vi "Insert Error.Record_New.vi"(7 "Code":string, 8 "error in (no error)":errorcluster, 9 "Source":string, 10 "Case":string, 11 "Model":string) -> (0 "error out":errorcluster)   [LabVIEW 2017, in "SQLite.lvclass"]
doc: "更新Limitation表格里面的Min和Max，根据输入的不同而更新不同的内容。\nValue 的输入必须最少包含Min和Max的值。\n\n2015-11-03 10:20:20\n蒋松\njiangsong@outlook.com"
uses:
  SQLite.lvclass
  SQLiteFileName.ctl
  TabelFullName.ctl
  <vilib>/Utility/error.llb/Trim Whitespace.vi
  <userlib>/sushu/sushu.lvlib
  <userlib>/LabSQL/LabSQL.lvlib
panel:
  in  "VI Ref":refnum<vi>
  in  "Alarm?":bool=TRUE
  in  "CMD":T1(ring)=enum."Read"
  out "concatenated string":string
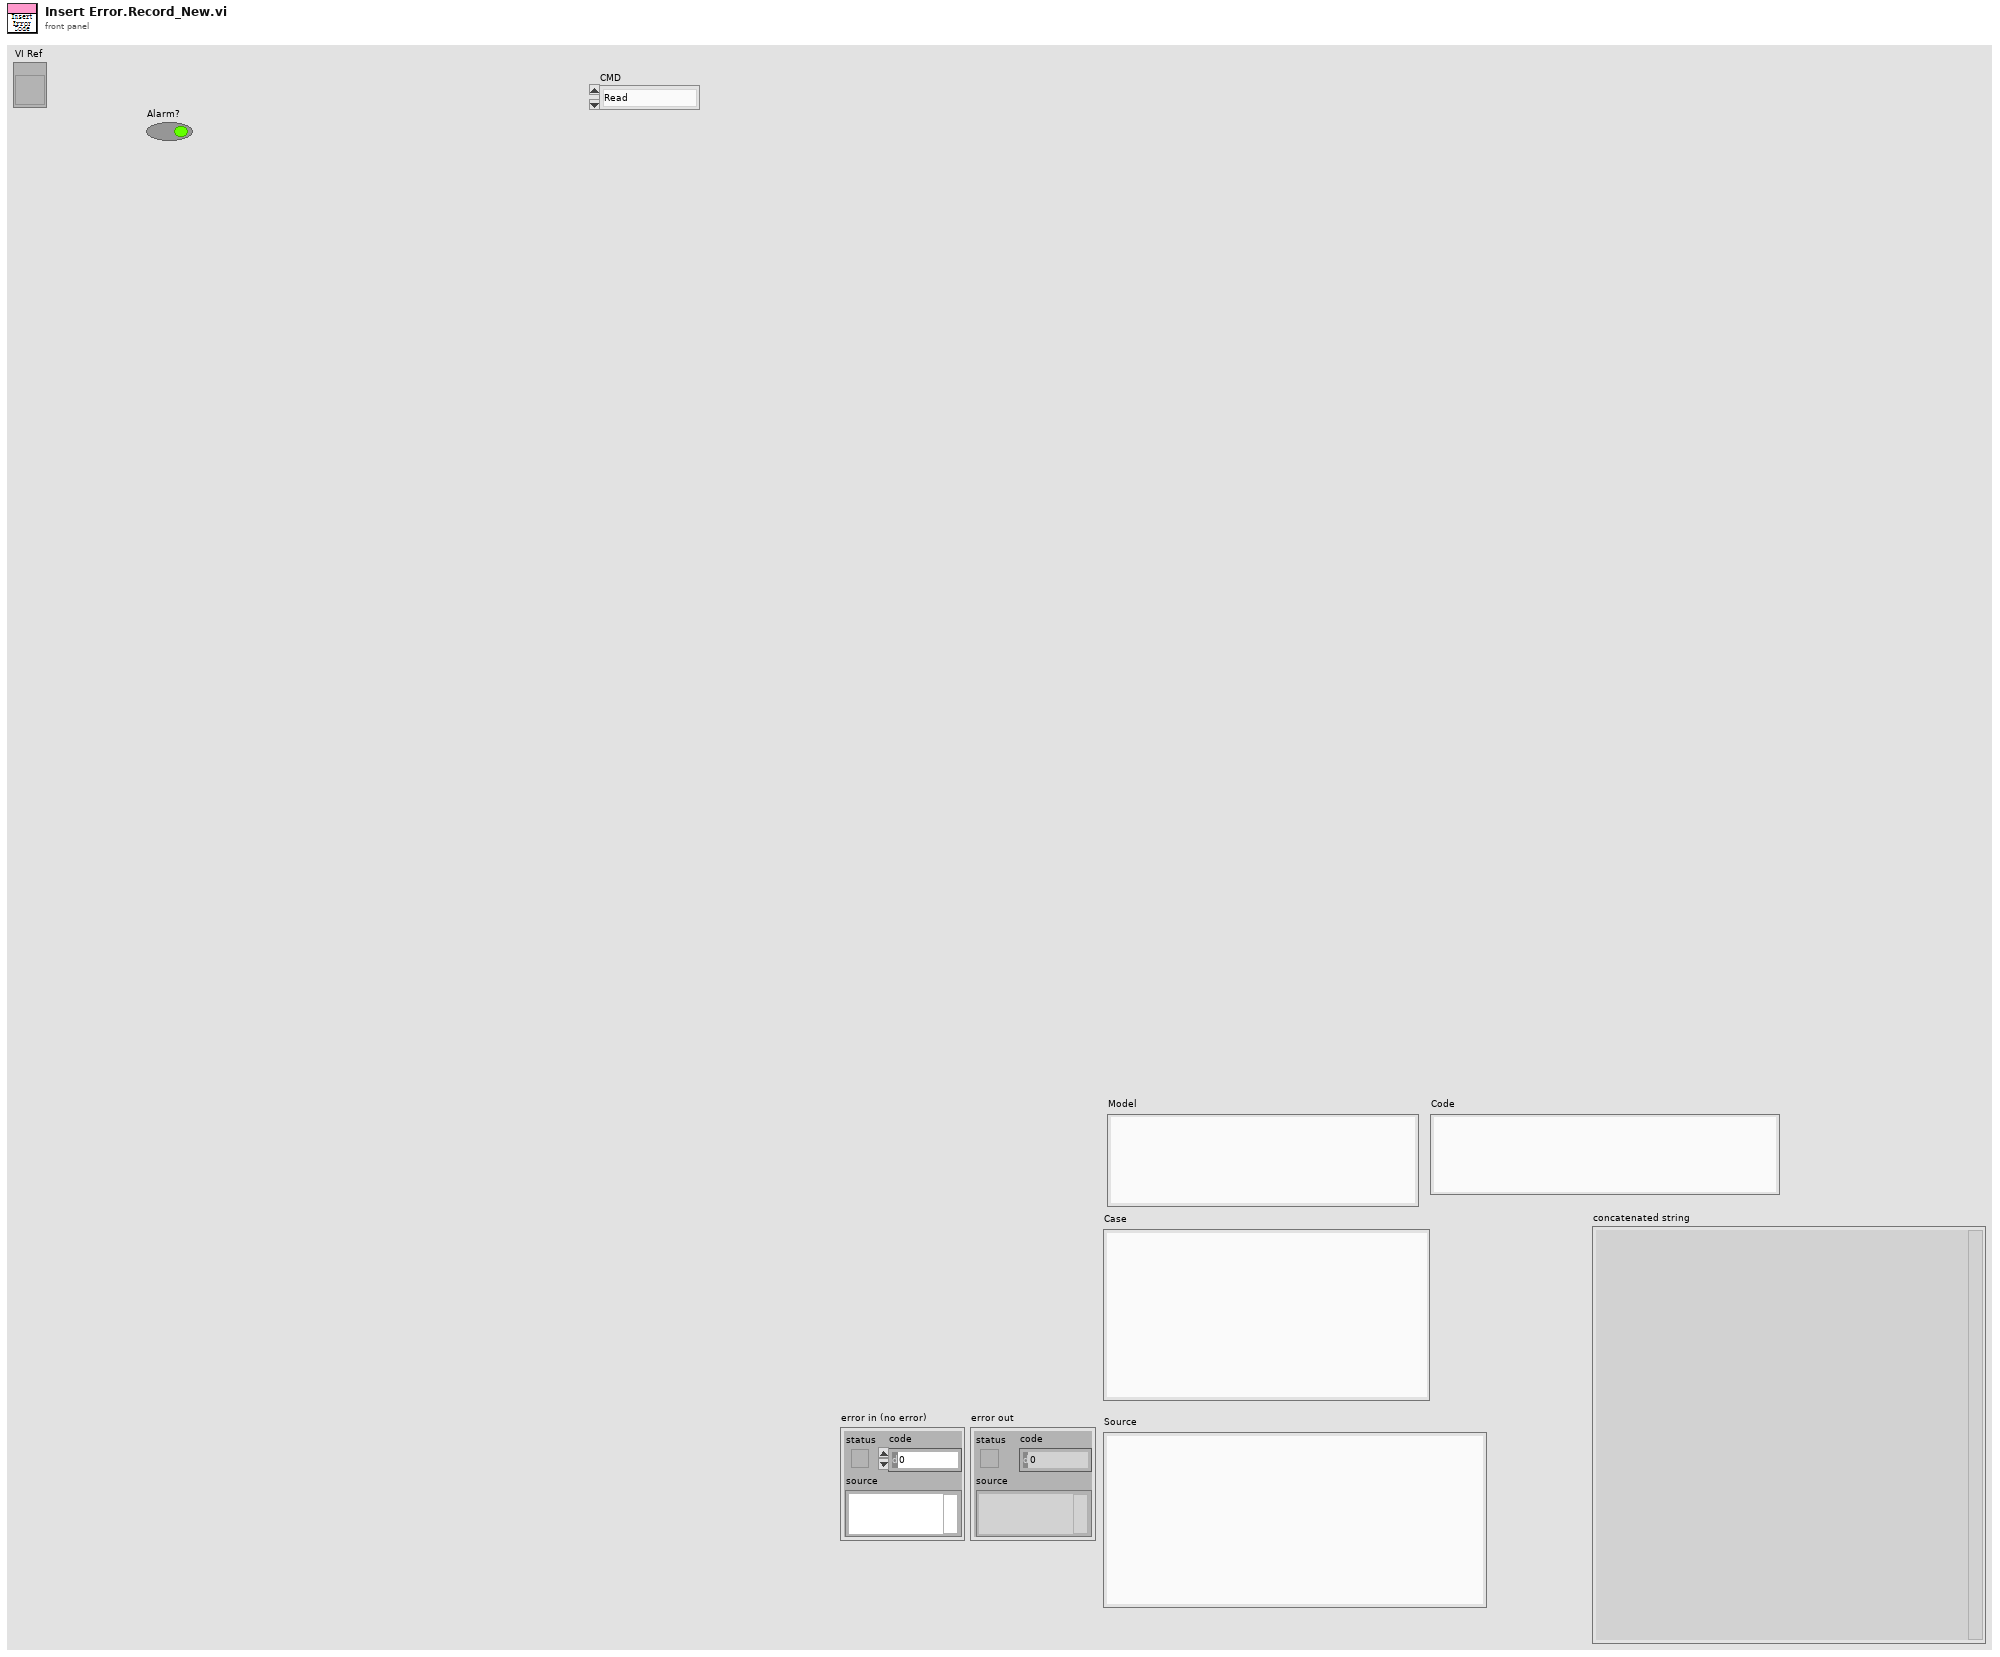
[diagram p1: front panel]
types:
  T1 = enum16{"Initialize", "Read", "Write", "UnInitialize"}
  T2 = typedef "SQLite.lvclass/TabelFullName.ctl" = string
  T3 = typedef "SQLite.lvclass/SQLiteFileName.ctl" = string
  T4 = cluster{"Current VI Reference":refnum<vi>, "Close Panel on Exit?":bool}
  T5 = cluster{"Core":cluster{"Current VI Reference":refnum<vi>, "Close Panel on Exit?":bool}, "VI Name":string}
  T6 = enum32{"invalid app kind", "Development System", "Run Time System", "Student Edition", "Embedded LabVIEW", "Evaluation", "Custom"}
  T7 = enum32{"Invalid", "Standard", "Closed", "Hidden", "Minimized", "Maximized"}
  T8 = enum16{"Other", "SQL2008", "SQLite", "Access", "MySQL"}
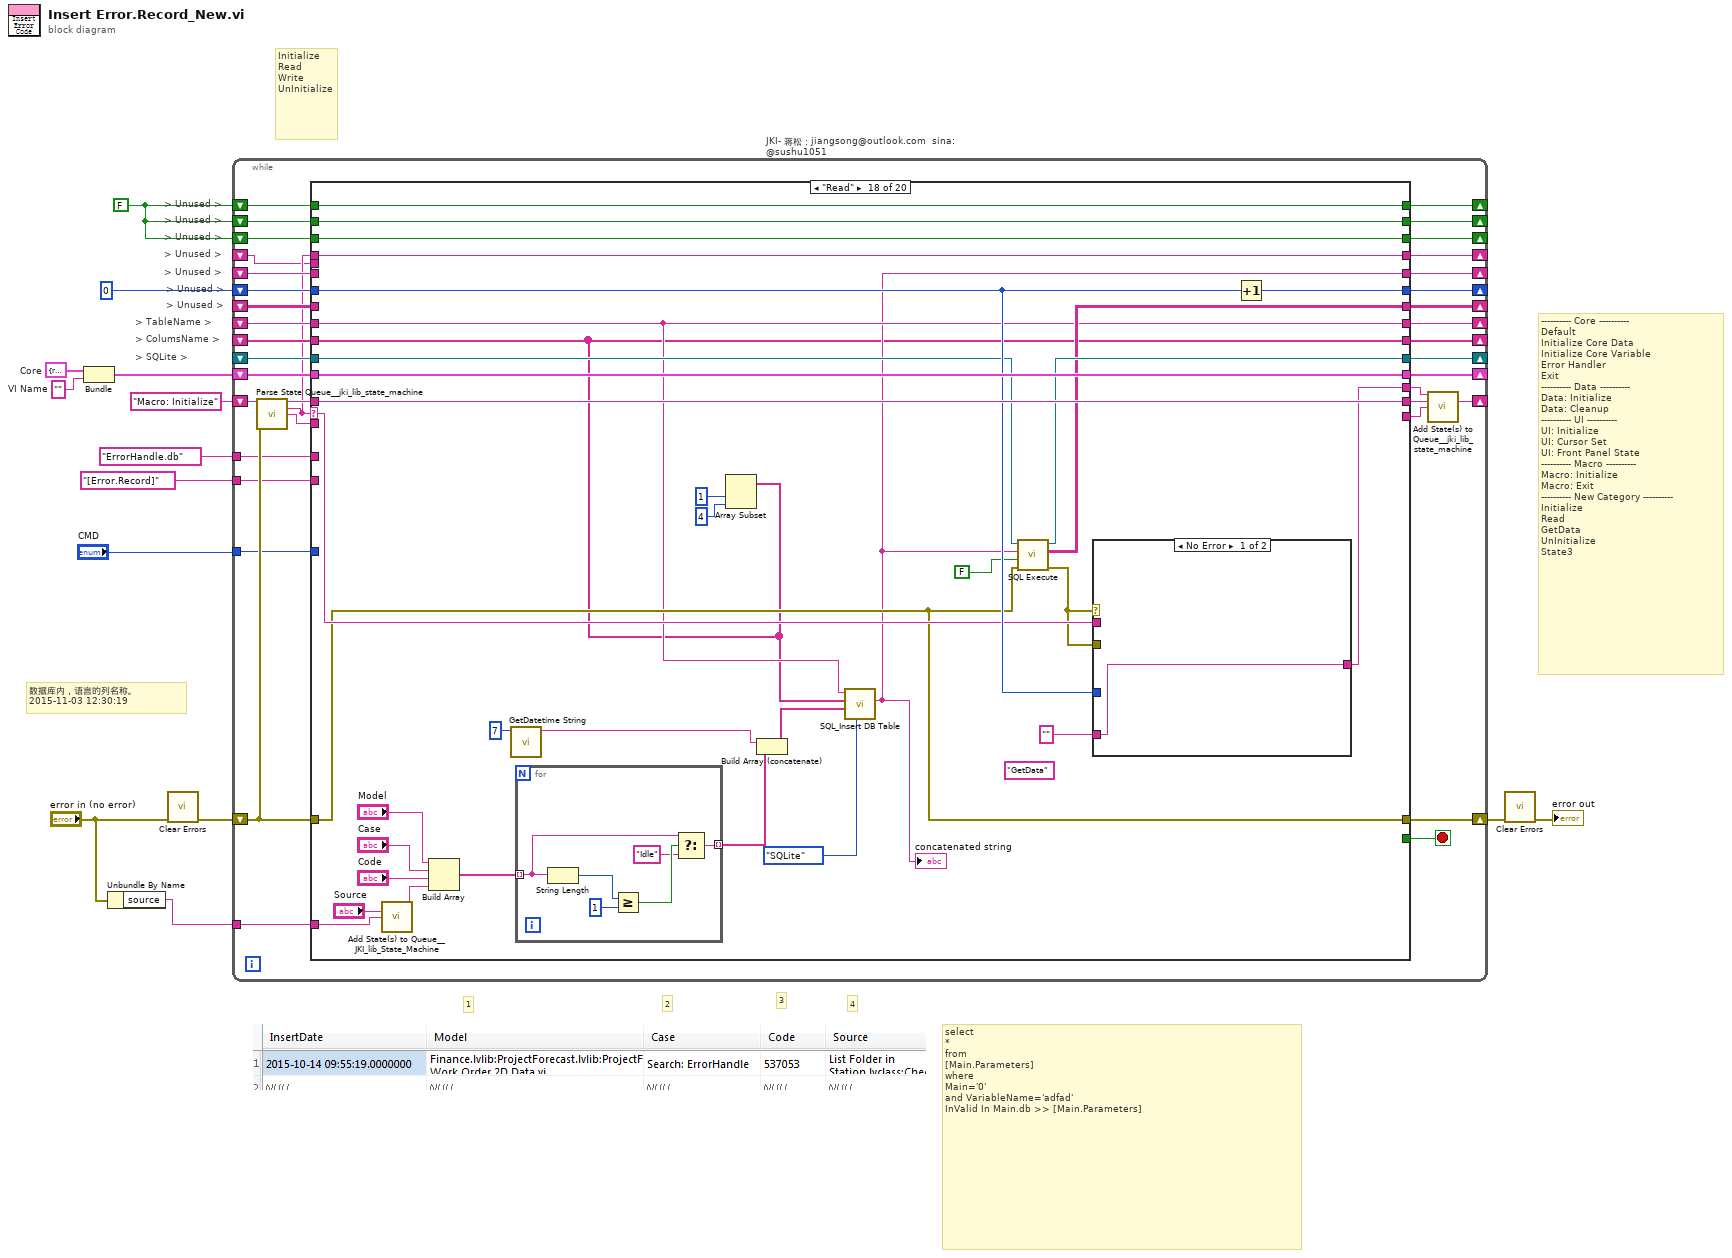
[diagram p0: block diagram]
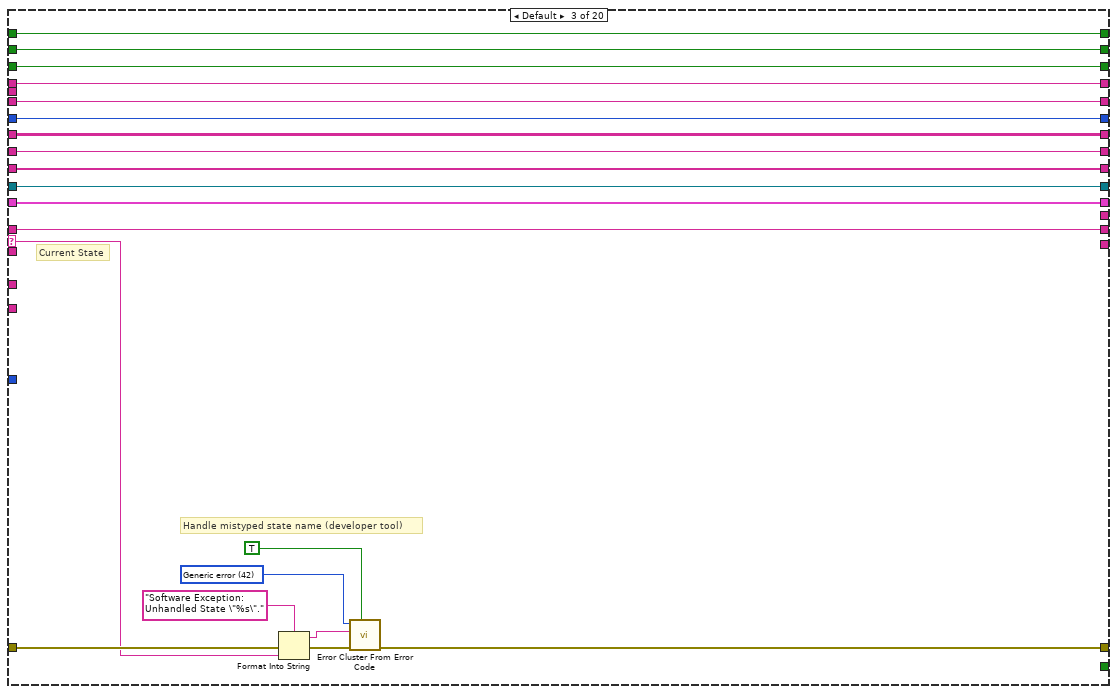
[diagram p4: hidden frame]
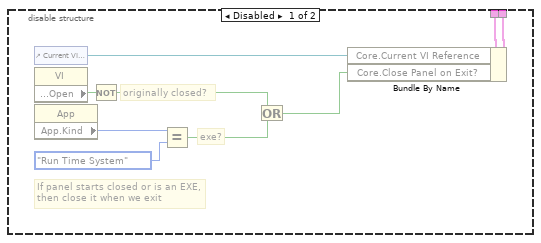
[diagram p6: hidden frame]
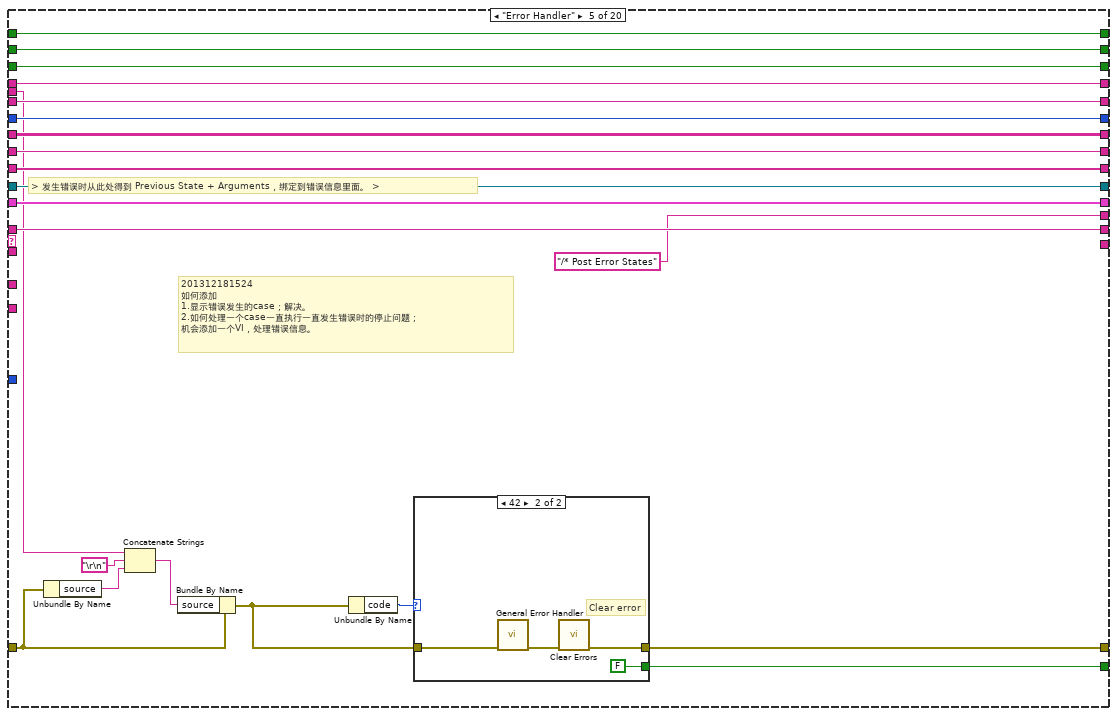
[diagram p7: hidden frame]
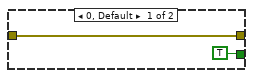
[diagram p8: hidden frame]
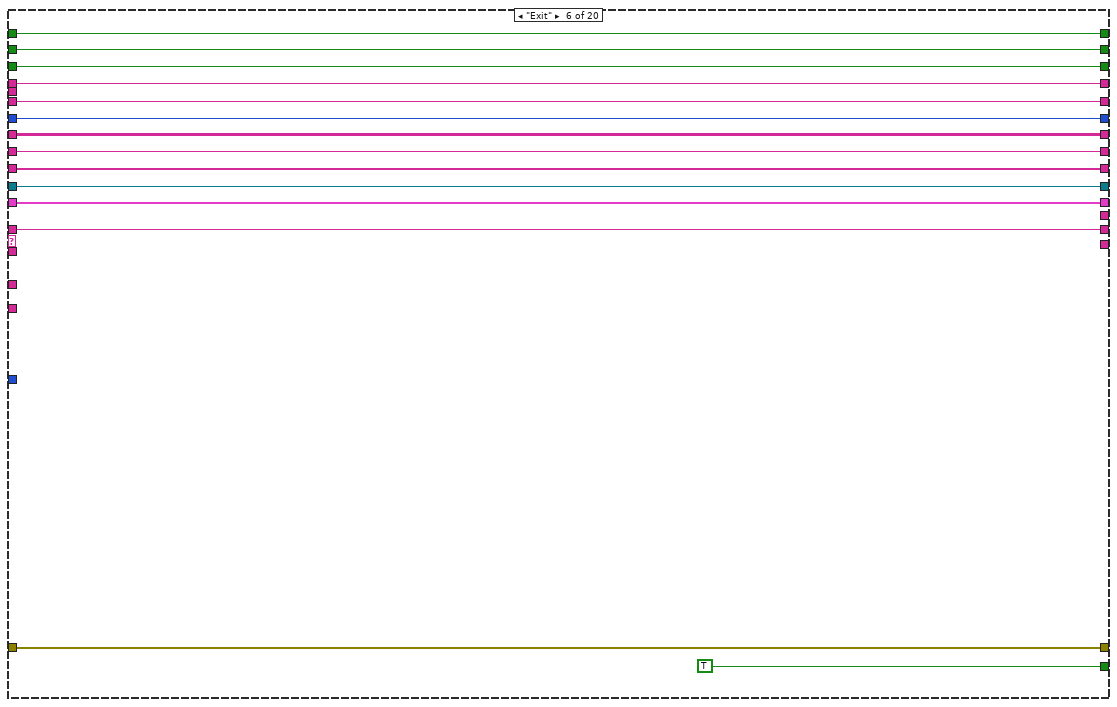
[diagram p9: hidden frame]
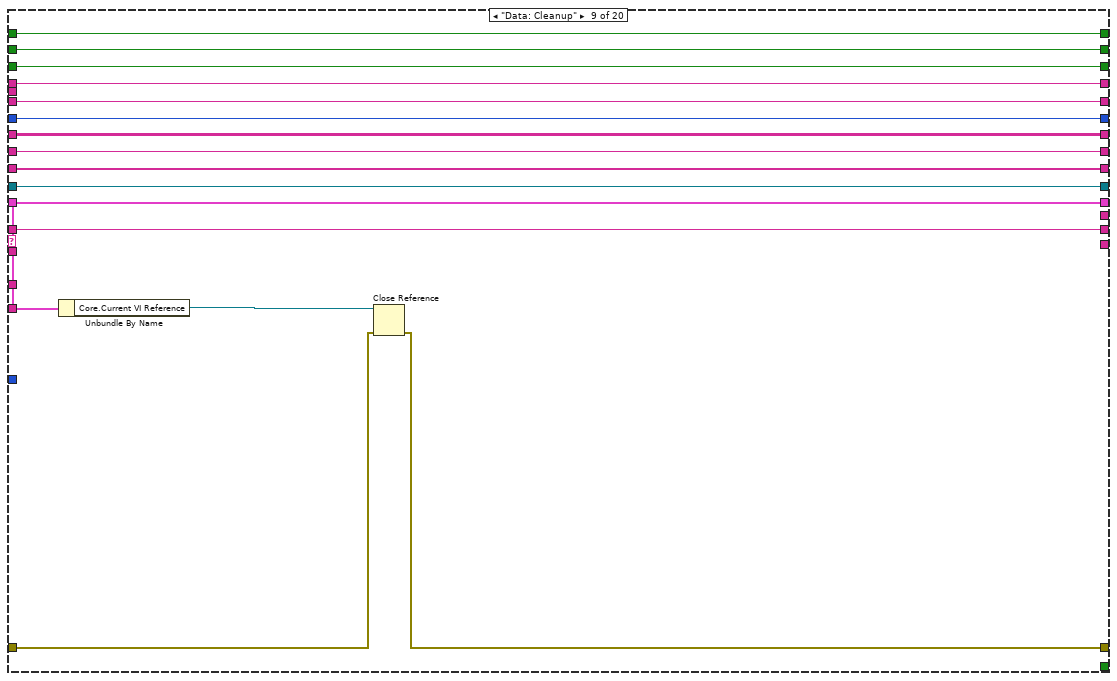
[diagram p12: hidden frame]
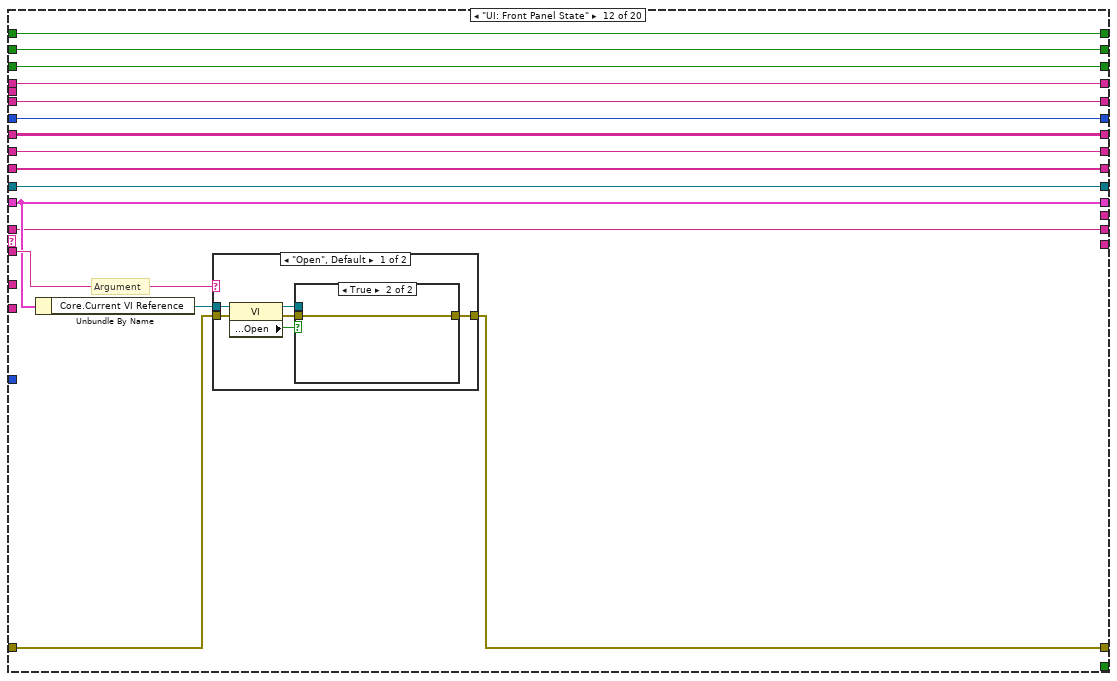
[diagram p15: hidden frame]
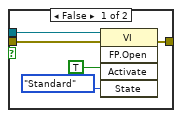
[diagram p16: hidden frame]
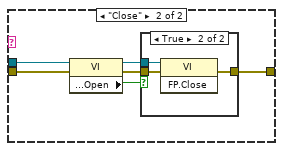
[diagram p17: hidden frame]
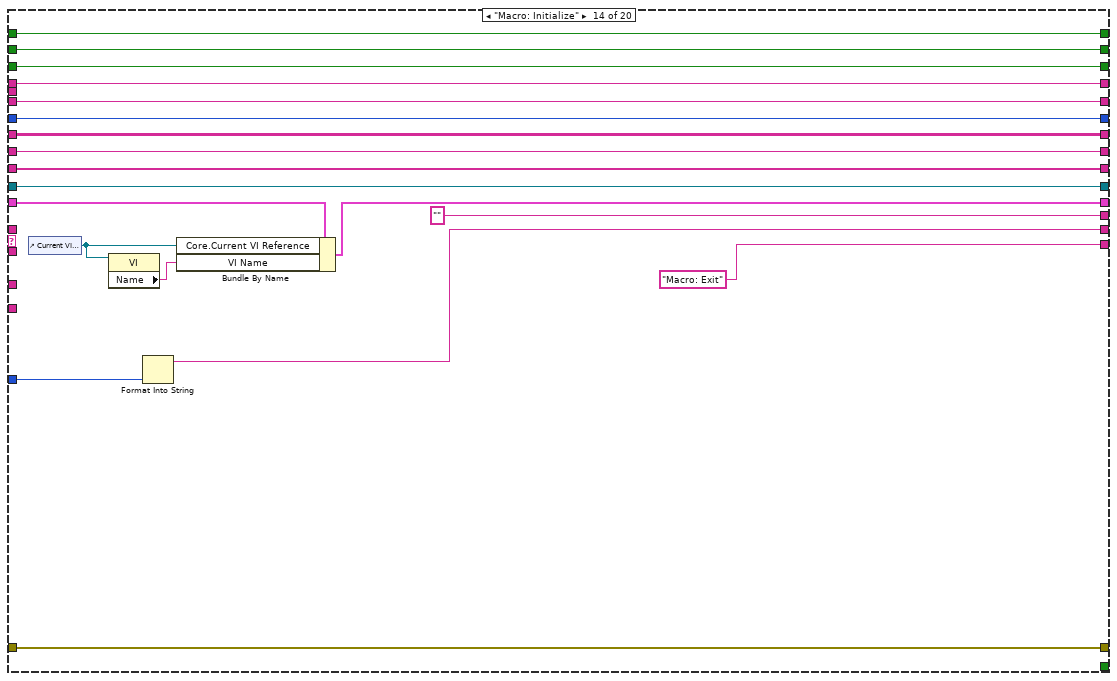
[diagram p20: hidden frame]
diagram:
  w14 = ""  # VI Name
  w13 = T4 {"Current VI Reference"=refnum, "Close Panel on Exit?"=FALSE}  # Core
  w8 = FALSE
  # "Initialize\nRead\nWrite\nUnInitialize"
  # "> Unused >"
  # "> Unused >"
  # "> Unused >"
  # "> Unused >"
  # "> Unused >"
  # "> Unused >"
  # "> SQLite >"
  # "> ColumsName >"
  # "> TableName >"
  # "> Unused >"
  # "---------- Core ----------\nDefault\nInitialize Core Data\nInitialize Core Variable\nError Handler\nExit\n---------- Data ----------\nData: Initialize\nData: Cleanup\n---------- UI ----------\nUI: Initialize\nUI: Cursor Set\nUI: Front Panel State\n---------- Macro ----------\nMacro: Initialize\nMacro: Exit\n---------- New Category ----------\nInitialize\nRead\nGetData\nUnInitialize\nState3"
  # "数据库内，语言的列名称。\n2015-11-03 12:30:19"
  # "4"
  # "3"
  # "2"
  # "1"
  # "select\n*\nfrom\n[Main.Parameters]\nwhere\nMain='0'\nand VariableName='adfad'\nInValid In Main.db >> [Main.Parameters]"
  n1 = Bundle("Core"=w13, "VI Name"=w14) -> (w12:T5)  [unwired: 1 in]
  n2 = Unbundle By Name("error in (no error)") -> ("source"=w2:string)
  n3 = call <vilib>:"Clear Errors.vi"("error in (no error)"="error in (no error)") -> ("error out"=w4:errorcluster)  [unwired: 5 in, 1 out]
  n4 = while "JKI- 蒋松：jiangsong@outlook.com  sina: @sushu1051" {
    shift-right: [w49] -> w5
    shift-left: w4 -> [w47]
    shift-right: [w36] -> _
    shift-left: "Macro: Initialize" -> [w37]
    shift-right: [w43] -> _
    shift-left: _ -> [w45]
    shift-right: [w44] -> _
    shift-left: _ -> [w46]
    shift-right: [w38] -> _
    shift-left: w12 -> [w41]
    shift-right: [w39] -> _
    shift-left: _ -> [w32]
    shift-right: [w40] -> _
    shift-left: _ -> [w42]
    shift-right: [w31] -> _
    shift-left: 0 -> [w30]
    shift-right: [w24] -> _
    shift-left: w8 -> [w22]
    shift-right: [w23] -> _
    shift-left: w8 -> [w21]
    shift-right: [w26] -> _
    shift-left: _ -> [w27]
    shift-right: [w25] -> _
    shift-left: _ -> [w16]
    shift-right: [w28] -> _
    shift-left: w8 -> [w29]
    tunnel: "CMD" -> [w20]
    tunnel: T3 "ErrorHandle.db" ("SQLiteFileName") -> [w19]
    tunnel: T2 "[Error.Record]" ("TabelFullName") -> [w18]
    tunnel: w2 -> [w15]
    stop <- w48 stop-if-true
    n5 = call <vilib>:"Parse State Queue__jki_lib_state_machine.vi"("State Queue"=w37, "Error In (no error)"=w47) -> ("Remaining States"=w51:string, "Current State"=w17:string, "Arguments"=w50:string)  [unwired: 10 in, 1 out]
    n6 = case shown="\"Read\"" w17 {
      selector: w17 -> [_ _ w85 _ _ _ _ _ _ _ _ _ _ _ _ _ _ w375 _ _]
      tunnel: w51 -> [w64 w71 w84 w104 w135 w156 w170 w184 w196 w211 w224 w237 w275 _ w308 w325 w351 w385 w421 w454]
      tunnel: w50 -> [_ _ _ _ _ _ _ _ _ _ _ w240 _ _ _ _ _ _ _ _]
      tunnel: [w63 w77 w86 w108 w129 w158 w172 w186 w198 w213 w226 w241 w277 w297 w315 w328 w332 w371 w406 w440] -> w49
      tunnel: w47 -> [w63 w77 w87 w108 w139 w158 w172 w186 w199 w213 w226 w242 w277 w297 w315 w328 w332 w371 w407 w441]
      tunnel: [w64 w71 w84 w104 w135 w156 w170 w184 w196 w211 w224 w237 w275 w283 w308 w325 w351 w385 w421 w454] -> w35
      tunnel: [_ _ _ _ w128 TRUE _ _ _ _ _ _ _ _ _ _ _ _ _ _] -> w48
      tunnel: w46 -> [w62 w76 w97 w111 w143 w163 w176 w189 w204 w217 w230 w246 w281 w300 w318 w331 w350 _ w408 w453]
      tunnel: w45 -> [w61 w75 w96 w110 w142 w162 w175 w188 w203 w216 w229 w245 w280 w299 w317 w330 _ w367 w420 w452]
      tunnel: [w62 w76 w97 w111 w143 w163 w176 w189 w204 w217 w230 w246 w281 w300 w318 w331 w350 w372 w408 w453] -> w44
      tunnel: [w61 w75 w96 w110 w142 w162 w175 w188 w203 w216 w229 w245 w280 w299 w317 w330 w333 w367 w420 w452] -> w43
      tunnel: w42 -> [w60 w74 w95 w109 w141 w161 w174 w187 w202 w215 w228 w244 w279 w298 w316 w329 _ w356 w419 w451]
      tunnel: w32 -> [w58 w72 w94 w105 w133 w157 w171 w185 w197 w212 w225 w238 w276 w296 w309 w326 _ w374 w418 w443]
      tunnel: w41 -> [w59 w73 w93 w107 w140 w160 w173 w177 w200 w214 w227 w239 w278 w285 w310 w327 w349 w384 w417 w450]
      tunnel: [w60 w74 w95 w109 w141 w161 w174 w187 w202 w215 w228 w244 w279 w298 w316 w329 w335 w356 w419 w451] -> w40
      tunnel: [w58 w72 w94 w105 w133 w157 w171 w185 w197 w212 w225 w238 w276 w296 w309 w326 w337 w373 w418 w442] -> w39
      tunnel: [w59 w73 w93 w106 w140 w160 w173 w177 w200 w214 w227 w239 w278 w284 w310 w327 w349 w384 w417 w450] -> w38
      tunnel: [_ _ _ _ "/* Post Error States" _ _ _ _ _ _ _ _ "" w307 _ _ w377 _ _] -> w34
      tunnel: [_ _ _ _ _ _ _ _ _ _ _ _ _ "Macro: Exit" _ _ _ _ _ _] -> w33
      tunnel: w30 -> [w57 w70 w83 w103 w132 w155 w169 w183 w195 w210 w223 w236 w274 w295 w306 w324 w348 w378 w416 w449]
      tunnel: [w57 w70 w83 w103 w132 w155 w169 w183 w195 w210 w223 w236 w274 w295 w306 w324 w348 w379 w416 w449] -> w31
      tunnel: w21 -> [w55 w68 w81 w101 w126 w153 w167 w181 w193 w208 w221 w234 w272 w291 w304 w322 w343 w382 w415 w448]
      tunnel: w22 -> [w54 w67 w80 w100 w125 w152 w166 w180 w192 w207 w220 w233 w271 w290 w303 w321 w344 w381 w414 w447]
      tunnel: [w55 w68 w81 w101 w126 w153 w167 w181 w193 w208 w221 w234 w272 w291 w304 w322 w343 w382 w415 w448] -> w23
      tunnel: [w54 w67 w80 w100 w125 w152 w166 w180 w192 w207 w220 w233 w271 w290 w303 w321 w344 w381 w414 w447] -> w24
      tunnel: w17 -> [w53 w66 w79 w99 w124 w151 w165 w179 w191 w206 w219 w232 w270 w289 w302 w320 w345 w380 w413 w446]
      tunnel: w27 -> [w52 w65 w78 w98 w123 w150 w164 w178 w190 w205 w218 w231 w269 w288 w301 w319 w346 _ w403 w445]
      tunnel: [w53 w66 w79 w99 w124 w151 w165 w179 w191 w206 w219 w232 w270 w289 w302 w320 w345 w380 w413 w446] -> w25
      tunnel: [w52 w65 w78 w98 w123 w150 w164 w178 w190 w205 w218 w231 w269 w288 w301 w319 w346 w366 w403 w445] -> w26
      tunnel: w29 -> [w56 w69 w82 w102 w127 w154 w168 w182 w194 w209 w222 w235 w273 w292 w305 w323 w347 w383 w412 w444]
      tunnel: [w56 w69 w82 w102 w127 w154 w168 w182 w194 w209 w222 w235 w273 w292 w305 w323 w347 w383 w412 w444] -> w28
      tunnel: w20 -> [_ _ _ _ _ _ _ _ _ _ _ _ _ w282 _ _ _ _ _ _]
      tunnel: w19 -> [_ _ _ _ _ _ _ _ _ _ _ _ _ _ _ _ w336 _ w405 _]
      tunnel: w18 -> [_ _ _ _ _ _ _ _ _ _ _ _ _ _ _ _ w334 _ w404 _]
      tunnel: w16 -> [_ _ _ _ w122 _ _ _ _ _ _ _ _ _ _ _ _ _ _ _]
      tunnel: w15 -> [_ _ _ _ _ _ _ _ _ _ _ _ _ _ _ _ _ w352 _ _]
      frame "Idle" {
      }
      frame "---------- Core ----------" {
      }
      frame Default {
        w89 = 42 items=["No error", "Argument error", "Memory is full", "Out of zone", "End of file", "File already open", "Generic file I/O error", "File not found", "File permission error", "Disk is full", "Duplicate path", "Too many files open", "System feature not enabled", "Resource file not found", "Cannot add resource", "Resource not found", "Image not found", "Image memory error", "Pen does not exist", "Config type invalid", "Config token not found", "Config parse error", "Config memory error", "Bad external code format", "Bad external code offset", "External code not present", "Null window", "Destroy window error", "Null menu", "Print aborted", "Bad print record", "Print driver error", "Windows error during printing", "Memory error during printing", "Print dialog error", "Generic print error", "Invalid device refnum", "Device not found", "Device parameter error", "Device unit error", "Cannot open device", "Device call aborted", "Generic error", "Cancelled by user", "Object ID too low", "Object ID too high", "Object not in heap", "Unknown heap", "Unknown object (invalid DefProc)", "Unknown object (DefProc not in table)", "Message out of range", "Invalid (null) method", "Unknown message", "Manager call not supported", "Bad address", "Network operation in progress", "Network operation timed out", "Connection is busy", "Network attribute not supported", "Network error", "Address in use", "System out of memory", "Connection aborted", "Connection refused", "Not connected", "Already connected", "Connection closed", "Initialization error (interapplication manager)", "Bad occurrence", "Wait on unbound occurrence handler", "Occurrence queue overflow", "Datalog type conflict", "Unused", "Unrecognized type (interapplication manager)", "Memory corrupt", "Failed to make temporary DLL", "Old CIN version", "Drag socket not found", "Failed to load drop-object", "Failed to register OLE object", "Failed to release OLE object", "Format specifier type mismatch", "Unknown format specifier", "Too few format specifiers", "Too many format specifiers", "Scan failed", "Newer CIN version", "Error converting to variant", "Runtime menu error", "Password tampered", "Variant attribute not found", "Incompatible variant data type", "Event data is not available", "Event Store is not present", "Occurrence is not found", "Event Queue is not created", "Event info is not available", "Refnum passed is NULL", "Error retrieving Class GUID", "Error retrieving CoClass GUID", "Error retrieving TypeLib GUID.", "Bad built application magic bytes.", "Specific driver is different from the specific driver associated with the Logical Name.", "There is no session opened to the class driver.", "Max Error", "MAX - Error with config objects", "MAX - Error loading configuration", "MAX - Group not supported"]
        # "Current State"
        # "Handle mistyped state name (developer tool)"
        n7 = Format Into String(format string="Software Exception: Unhandled State \"%s\"." ("message"), error in=w87, w85) -> (resulting string=w90:string, error out=w91:errorcluster)  [unwired: 1 in]
        n8 = call <vilib>:"Error Cluster From Error Code.vi"("show call chain? (False)"=TRUE, "error in (no error)"=w91, "error message (\"\")"=w90, "error code (0)"=w89) -> ("error out"=w86:errorcluster)  [unwired: 5 in]
      }
      frame "Initialize Core Data" {
        n9 = disable-structure shown="Enabled" {
          disable-tunnel: w107 -> [w113 w121]
          disable-tunnel: [w112 w121] -> w106
          frame Disabled {
            # "originally closed?"
            # "exe?"
            # "If panel starts closed or is an EXE, then close it when we exit"
            n10 = control-ref of="Current VI Reference"() -> (w120:refnum<vi>)
            n11 = property class="VI"() -> ("Front Panel.Open"=w114:bool)  [unwired: 2 in, 2 out]
            n12 = property class="App"() -> ("App.Kind"=w115:T6)  [unwired: 2 in, 2 out]
            n13 = Not(x=w114) -> (.not. x?=w117:bool)
            n14 = Equal?(x=w115, y=T6."Run Time System" ("Application:Kind")) -> (x = y?=w118:bool)
            n15 = Or(x=w117, y=w118) -> (x .or. y?=w119:bool)
            n16 = Bundle By Name(cluster=w113, "Core.Current VI Reference"=w120, "Core.Close Panel on Exit?"=w119) -> (w112:T5)
          }
          frame Enabled {
          }
        }
      }
      frame "Error Handler" {
        # "> 发生错误时从此处得到 Previous State + Arguments，绑定到错误信息里面。 >"
        # "201312181524\n如何添加\n1.显示错误发生的case；解决。\n2.如何处理一个case一直执行一直发生错误时的停止问题；\n机会添加一个VI，处理错误信息。"
        # "Clear error"
        n17 = Unbundle By Name(w139) -> ("source"=w137:string)
        n18 = Concatenate Strings(w122, "\r\n", w137) -> (w136:string)
        n19 = Bundle By Name(cluster=w139, "source"=w136) -> (w130:errorcluster)
        n20 = Unbundle By Name(w130) -> ("code"=w131:i32)
        n21 = case shown="42" w131 {
          tunnel: [TRUE FALSE] -> w128
          tunnel: w130 -> [w145 w148]
          tunnel: [w145 w146] -> w129
          frame 0, Default {
          }
          frame 42 {
            n22 = call <vilib>:"General Error Handler.vi"("error in (no error)"=w148) -> ("error out"=w147:errorcluster)  [unwired: 10 in, 4 out]
            n23 = call <vilib>:"Clear Errors.vi"("error in (no error)"=w147) -> ("error out"=w146:errorcluster)  [unwired: 5 in, 1 out]
          }
        }
      }
      frame "Exit" {
      }
      frame "---------- Data ----------" {
      }
      frame "Data: Initialize" {
      }
      frame "Data: Cleanup" {
        n24 = Unbundle By Name(w200) -> ("Core.Current VI Reference"=w201:refnum<vi>)
        n25 = Close Reference(reference=w201, error in (no error)=w199) -> (error out=w198:errorcluster)
      }
      frame "---------- UI ----------" {
      }
      frame "UI: Initialize" {
      }
      frame "UI: Front Panel State" {
        # "Argument"
        n26 = Unbundle By Name(w239) -> ("Core.Current VI Reference"=w243:refnum<vi>)
        n27 = case shown="\"Open\", Default" w240 {
          tunnel: w242 -> [w250 w263]
          tunnel: [w252 w264] -> w241
          tunnel: w243 -> [w251 w261]
          frame "Open", Default {
            n28 = property class="VI"(reference=w251, error in=w250) -> (reference out=w248:refnum<vi>, error out=w249:errorcluster, "Front Panel.Open"=w247:bool)
            n29 = case shown="True" w247 {
              tunnel: [w255 w258] -> w252
              tunnel: w249 -> [w254 w258]
              tunnel: w248 -> [w253 _]
              frame False {
                n30 = invoke class="VI" method="FP.Open"(reference=w253, error in=w254, "Activate"=TRUE, "State"=T7."Standard") -> (error out=w255:errorcluster)  [unwired: 1 in, 4 out]
              }
              frame True {
              }
            }
          }
          frame "Close" {
            n31 = property class="VI"(reference=w261, error in=w263) -> (reference out=w260:refnum<vi>, error out=w262:errorcluster, "Front Panel.Open"=w259:bool)
            n32 = case shown="True" w259 {
              tunnel: [w265 w268] -> w264
              tunnel: w262 -> [w265 w267]
              tunnel: w260 -> [_ w266]
              frame False {
              }
              frame True {
                n33 = invoke class="VI" method="FP.Close"(reference=w266, error in=w267) -> (error out=w268:errorcluster)  [unwired: 1 in, 2 out]
              }
            }
          }
        }
      }
      frame "---------- Macro ----------" {
      }
      frame "Macro: Initialize" {
        n34 = control-ref of="Current VI Reference"() -> (w286:refnum<vi>)
        n35 = property class="VI"(reference=w286) -> ("Name"=w287:string)  [unwired: 1 in, 2 out]
        n36 = Format Into String(w282) -> (resulting string=w283:string)  [unwired: 3 in, 1 out]
        n37 = Bundle By Name(cluster=w285, "Core.Current VI Reference"=w286, "VI Name"=w287) -> (w284:T5)
      }
      frame "Macro: Exit" {
        n38 = Unbundle By Name(w310) -> ("Core.Close Panel on Exit?"=w311:bool)
        n39 = Select(t="UI: Front Panel State >> Close", s=w311, f="") -> ()  [unwired: 1 out]
        n40 = call <vilib>:"Add State(s) to Queue__jki_lib_state_machine.vi"("State(s) at Back (\"\")"="Data: Cleanup\nExit") -> ("States Out"=w307:string)  [unwired: 14 in]
      }
      frame "---------- New Category ----------" {
      }
      frame "Initialize" {
        n41 = Concatenate Strings(w334) -> (w333:string)
        n42 = call "SQLite File Path.vi"("SQLiteFileName"=w336, "SQLite in"=refnum<class "SQLite.lvclass"> refnum ("SQLite.lvclass")) -> ("string"=w340:string, "SQLite out"=w342:refnum<class "SQLite.lvclass">)  [unwired: 7 in, 1 out]
        n43 = call-dynamic "Open Connection.vi"("ConnectionString"=w340, "HostDB in"=w342) -> ("error out"=w339:errorcluster, "HostDB out"=w338:refnum<class "SQLite.lvclass">)  [unwired: 8 in]
        n44 = call-dynamic "Get Table Columns Name.vi"("error in (no error)"=w339, "TableName"=w333, "HostDB in"=w338) -> ("Table_ColunmsList"=w335:string[], "HostDB out"=w337:refnum<class "SQLite.lvclass">)  [unwired: 3 in, 4 out]
      }
      frame "Read" {
        (unwired) "GetData" ("f")
        n45 = call <vilib>:"Add State(s) to Queue__JKI_lib_State_Machine.vi"("State(s) in (\"\")"="Source", "State(s) at Back (\"\")"=w352) -> ("States Out"=w353:string)  [unwired: 13 in]
        n46 = Build Array("Model", "Case", "Code", w353) -> (w359:string[])
        n47 = call <userlib>:"GetDatetime String.vi"("u?"=7) -> ("date/time string"=w354:string)  [unwired: 6 in, 4 out]
        n48 = for {
          tunnel: w359 -> [w388] mode=indexing
          tunnel: [w386] -> w358 mode=indexing
          n49 = String Length(string=w388) -> (length=w391:i32)
          n50 = Greater Or Equal?(x=w391, y=1) -> (x >= y?=w389:bool)
          n51 = Select(t=w388, s=w389, f="Idle") -> (s? t:f=w386:string)
        }
        n52 = Array Subset(array=w356, index=1, length=4) -> ()  [unwired: 1 out]
        n53 = Build Array (concatenate)(w354, w358) -> (w355:string[])
        n54 = call <userlib>:"SQL_Insert DB Table.vi"("DB Type"=T8."SQLite", "ColumnsValue"=w355, "ColumnsName"=w356, "Table Name"=w367) -> ("Insert DB String"=w366:string)  [unwired: 7 in]
        "concatenated string" <- w366
        n55 = call-dynamic "SQL Execute.vi"("error in (no error)"=w371, "Return Data (T)"=FALSE, "Command Text"=w366, "HostDB in"=w374) -> ("error out"=w370:errorcluster, "Table Control"=w372:string[][], "HostDB out"=w373:refnum<class "SQLite.lvclass">)  [unwired: 3 in, 2 out]
        n56 = case shown="No Error" w370 {
          tunnel: w370 -> [_ w402]
          tunnel: w378 -> [_ w401]
          tunnel: [w392 w398] -> w377
          tunnel: "" ("f") -> [w392 w397]
          tunnel: w375 -> [_ w394]
          frame No Error {
          }
          frame Error {
            n57 = Unbundle By Name(w402) -> ("status"=w393:bool)
            n58 = Equal To 0?(x=w401) -> (x = 0?=w400:bool)
            n59 = And(x=w393, y=w400) -> (x .and. y?=w399:bool)
            n60 = call <vilib>:"Add State(s) to Queue__jki_lib_state_machine.vi"("State(s) in Front (\"\")"="Initialize" ("Remaining States"), "State(s) in (\"\")"=w394) -> ("States Out"=w395:string)  [unwired: 13 in]
            n61 = Select(t=w395, s=w399, f=w397) -> (s? t:f=w398:string)
          }
        }
        n62 = Increment(x=w378) -> (x+1=w379:i32)
      }
      frame "GetData" {
        n63 = Empty Array?(array=w408) -> (empty?=w410:bool)
        n64 = And(x=w410, y="Alarm?") -> (x .and. y?=w411:bool)
        n65 = case shown="False" w411 {
          tunnel: [w425 w438] -> w406
          tunnel: w407 -> [w425 w439]
          tunnel: w403 -> [_ w435]
          tunnel: w405 -> [_ w437]
          tunnel: w404 -> [_ w436]
          tunnel: w408 -> [w422 _]
          frame False {
            w423 = 0 ("index (row)")
            # "DBL 和 字符串 都输出，需要那个用那个。\n2015-11-03 10:44:12\n蒋松"
            n66 = Index Array(array=w422, index (row)=w423, index (col)=w423) -> ()  [unwired: 1 out]
            n67 = Index Array(array=w422, index (col)=0 ("disabled index (col)")) -> ()  [unwired: 1 in, 1 out]
          }
          frame True {
            n68 = Concatenate Strings(w437) -> (w434:string)
            n69 = Concatenate Strings(w436) -> (w433:string)
            n70 = call <vilib>:"Build State String with Arguments__JKI_lib_State_Machine.vi"("Arguments (\"\")"=w433, "State"=w434) -> ("State with Arguments"=w431:string)  [unwired: 4 in]
            n71 = Concatenate Strings(w435, "InValid In " ("Message"), w431) -> (w430:string)
            n72 = call <userlib>:"Errors Handle Dialoge.vi"("VI Ref"="VI Ref", "Cancel Text"="Ignore", "OK Text"="OK", "error in (no error)"=w439, "Title Text"="Select VariableName!", "Message"=w430) -> ("error out"=w438:errorcluster)  [unwired: 4 in, 1 out]
          }
        }
      }
      frame "UnInitialize" {
        n73 = call-dynamic "Close Connection.vi"("error in (no error)"=w441, "HostDB in"=w443) -> ("error out"=w440:errorcluster, "HostDB out"=w442:refnum<class "SQLite.lvclass">)  [unwired: 8 in]
      }
    }
    n74 = call <vilib>:"Add State(s) to Queue__jki_lib_state_machine.vi"("State(s) in Front (\"\")"=w34, "State(s) in (\"\")"=w35, "State(s) at Back (\"\")"=w33) -> ("States Out"=w36:string)  [unwired: 12 in]
  }
  n75 = call <vilib>:"Clear Errors.vi"("error in (no error)"=w5) -> ("error out"=→"error out":errorcluster)  [unwired: 5 in, 1 out]
